vi "CheckIntercept.vi"(8 "error in (no error)":errorcluster, 10 "Game":refnum<class "Game.lvclass">, 11 "object in":refnum<class "PrimaryAttackerRole_v2.lvclass">) -> (0 "error out":errorcluster, 2 "intercepted":bool, 3 "object out":refnum<class "PrimaryAttackerRole_v2.lvclass">)   [LabVIEW 2023, in "PrimaryAttackerRole_v2.lvclass"]
uses:
  PrimaryAttackerRole_v2.lvclass
  Game_class/Game.lvclass
  Game_class/Game.lvclass/Game.ctl
  Events_class/Events.lvclass/Events.ctl
  Ball_class/Ball.lvclass/Ball.ctl
  Game_class/Read EventsRef.vi
  Game_class/Read BallRef.vi
  Ball_class/Read velocityNorm.vi
  Events_class/Read touch.vi
  Events_class/Read kick.vi
  <vilib>/Analysis/_algsub.llb/Vector Norm.vi
  <vilib>/Analysis/_algsub.llb/Real Vector Norm.vi
  Events_class/Events.lvclass
  Ball_class/Ball.lvclass
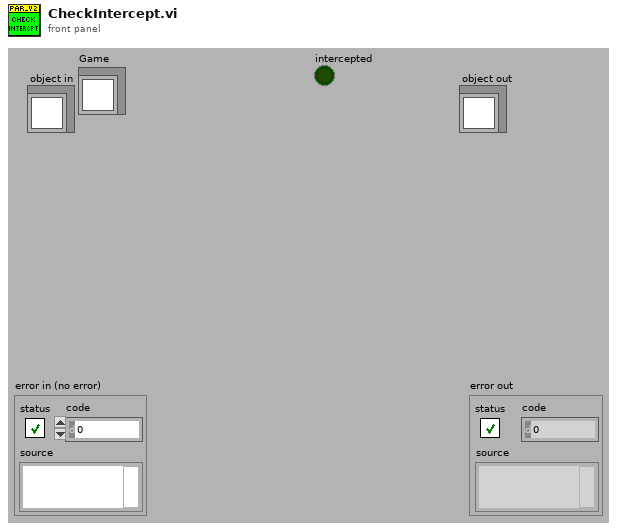
[diagram p1: front panel]
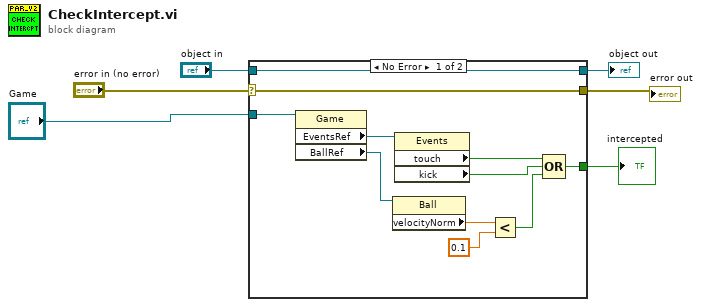
[diagram p0: block diagram]
diagram:
  n1 = case shown="No Error" "error in (no error)" {
    selector: "error in (no error)" -> [w17 w19]
    tunnel: [w17 w19] -> w5
    tunnel: [w16 w18] -> w3
    tunnel: "object in" -> [w16 w18]
    tunnel: "Game" -> [w15 _]
    tunnel: [w7 _] -> w2
    frame No Error {
      n2 = property class="Game"(reference=w15) -> ("EventsRef"=w14:refnum<class "Events.lvclass">, "BallRef"=w13:refnum<class "Ball.lvclass">)  [unwired: 1 in, 2 out]
      n3 = property class="Ball"(reference=w13) -> ("velocityNorm"=w12:dbl)  [unwired: 1 in, 2 out]
      n4 = property class="Events"(reference=w14) -> ("touch"=w10:bool, "kick"=w9:bool)  [unwired: 1 in, 2 out]
      n5 = Less?(x=w12, y=0.1) -> (x < y?=w8:bool)
      n6 = Compound Arithmetic op=OR(w10, w9, w8) -> (w7:bool)
    }
    frame Error {
    }
  }
  "error out" <- w5
  "object out" <- w3
  "intercepted" <- w2
